vi "Review Fiducials Dialog.vi"(7 "Console Log in":refnum<class "Console Log.lvclass">, 8 "error in":errorcluster, 11 "Potting Procedure in":refnum<class "Potting Procedure.lvclass">) -> (0 "error out":errorcluster, 2 "Canceled":bool, 3 "Potting Procedure out":refnum<class "Potting Procedure.lvclass">, 5 "Console Log out":refnum<class "Console Log.lvclass">)   [LabVIEW 2011]
uses:
  Procedure Classes/Potting Procedure/Potting Procedure.lvclass
  Application Utilities/Console Log/Console Log.lvclass
  Shared Components/Utils/Type Definitions/Fiducial with Source.ctl
  Shared Components/Vec3d Class/Vec3d Class.lvclass
  Shared Components/WorkTable Class/Type Definitions/Worktable_Mode.ctl
  Procedure Classes/Potting Procedure/Type Definitions/Inspect Fiducials.ctl
  Shared Components/Utils/Type Definitions/Fiducial Image.ctl
  Shared Components/Utils/Type Definitions/Physical Image.ctl
  <vilib>/vision/Image Controls.llb/IMAQ Image.ctl
  Procedure Classes/Potting Procedure/Type Definitions/Review Fiducials.ctl
panel:
  in  "reacquire BBM BR":bool
  in  "reacquire BBM TR":bool
  in  "reacquire BBM BL":bool
  in  "reacquire BBM TL":bool
  in  "reacquire HDI BR":bool
  in  "reacquire HDI TR":bool
  in  "reacquire HDI BL":bool
  in  "reacquire HDI TL":bool
  out "BBM BL View":T1(plugin-control)
  out "BBM BR View":T1(plugin-control)
  out "BBM TL View":T1(plugin-control)
  out "BBM TR View":T1(plugin-control)
  in  "idx":i32
  out "idx_label":string="1/10"
  out "Current Module":cluster{"Chuck":i32, "Slot":i32}={"Chuck"=1, "Slot"=1}
  in  "Previous":bool
  in  "Next":bool
  out "HDI BL View":T1(plugin-control)
  out "HDI BR View":T1(plugin-control)
  out "HDI TL View":T1(plugin-control)
  out "HDI TR View":T1(plugin-control)
  in  "OK Button":bool
  in  "Cancel Button":bool
  # "Pattern Recognition"
  # "Error"
  # "Click on images to correct fiducial positions.\nAll error fiducials must be corrected before continuing."
  # "User Defined"
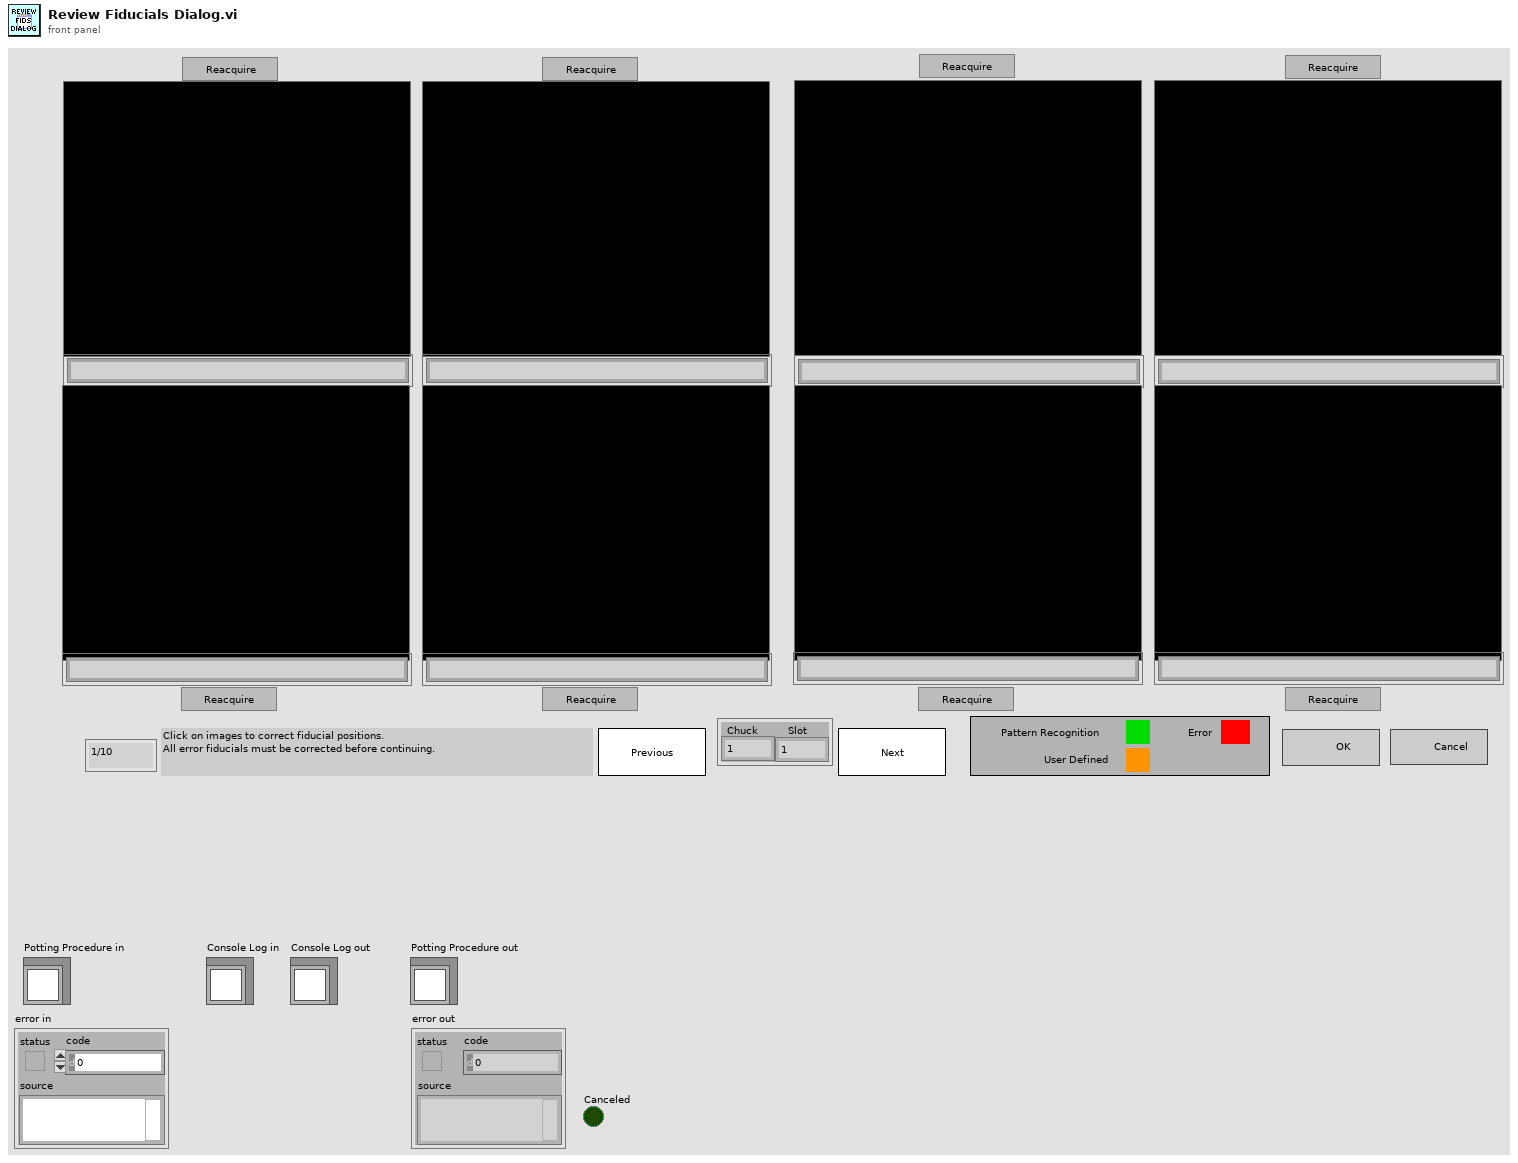
[diagram p1: front panel]
types:
  T1 = typedef "IMAQ Image.ctl" = refnum<image>
  T2 = typedef "Inspect Fiducials.ctl" = cluster{"Has Been Run?":bool, "Module-Chuck Fiducials":cluster{"Fiducials-HDI":T3[], "Fiducials-BBM":T3[], "Chuck":i32, "Slot":i32}[]}
  T3 = typedef "Fiducial Image.ctl" = cluster{"Fiducial Image":T4, "Selected Fiducial":T5, "fiducial name":string}
  T4 = typedef "Physical Image.ctl" = cluster{"Image Position":refnum<class "Vec3d Class.lvclass">, "Image Reference":T1, "Field of View":cluster{"x(mm)":dbl, "y(mm)":dbl}}
  T5 = typedef "Fiducial with Source.ctl" = cluster{"Fiducial Image Coordinate":refnum<class "Vec3d Class.lvclass">, "Fiducial Source":enum16{"Pattern Recognition", "User", "Error", "Default"}}
  T6 = cluster{"Fiducials-HDI":T3[], "Fiducials-BBM":T3[], "Chuck":i32, "Slot":i32}[]
  T7 = enum16{"None", "glue_resevoir_chuck", "stamp_tool_chuck", "weight_tool_chuck", "hdi_chuck_04"}
  T8 = typedef "Worktable_Mode.ctl" = enum16{"Encapsulation", "Gluing"}
  T9 = cluster{"Fiducials-HDI":T3[], "Fiducials-BBM":T3[], "Chuck":i32, "Slot":i32}
  T10 = enum16{"Pattern Recognition", "User", "Error", "Default"}
  T11 = typedef "LVPoint32TypeDef.ctl" = cluster{"Horizontal":i32, "Vertical":i32}
  T12 = typedef "Review Fiducials.ctl" = cluster{"Has Been Run?":bool}
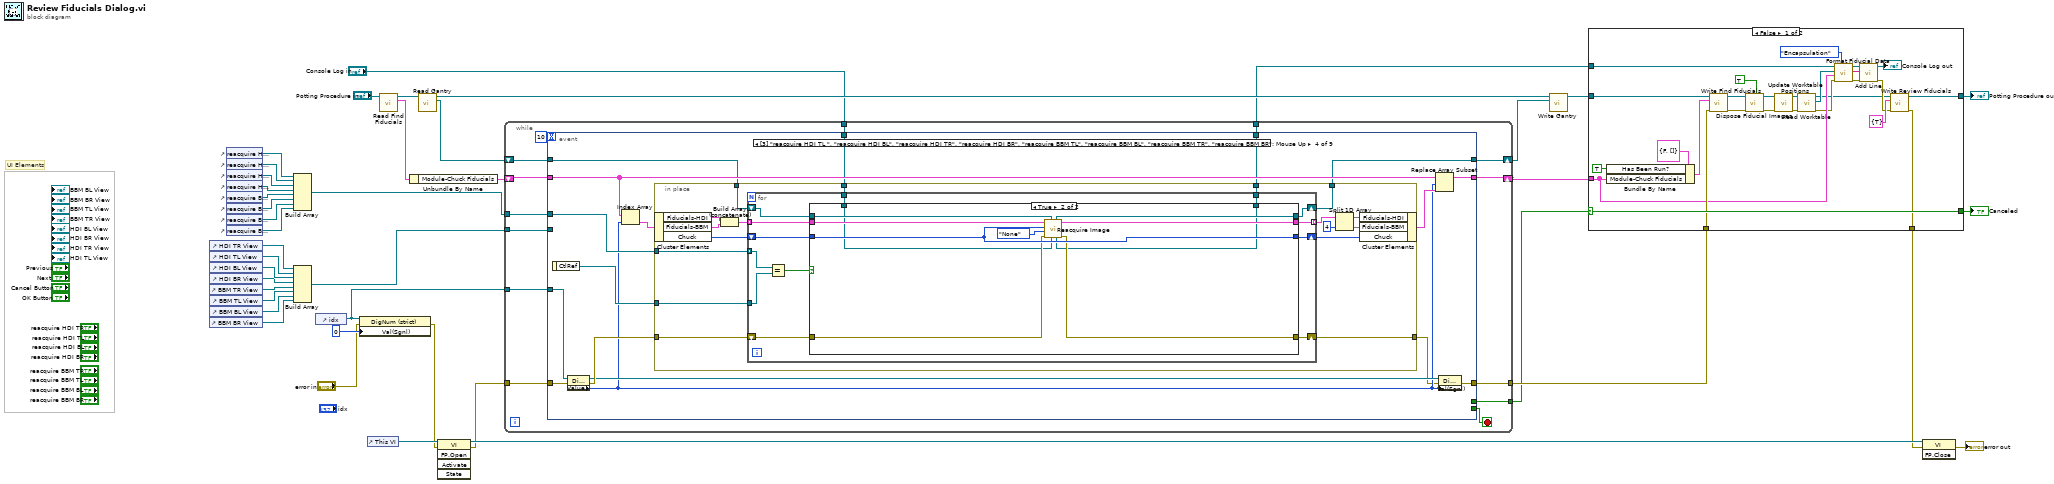
[diagram p0: block diagram]
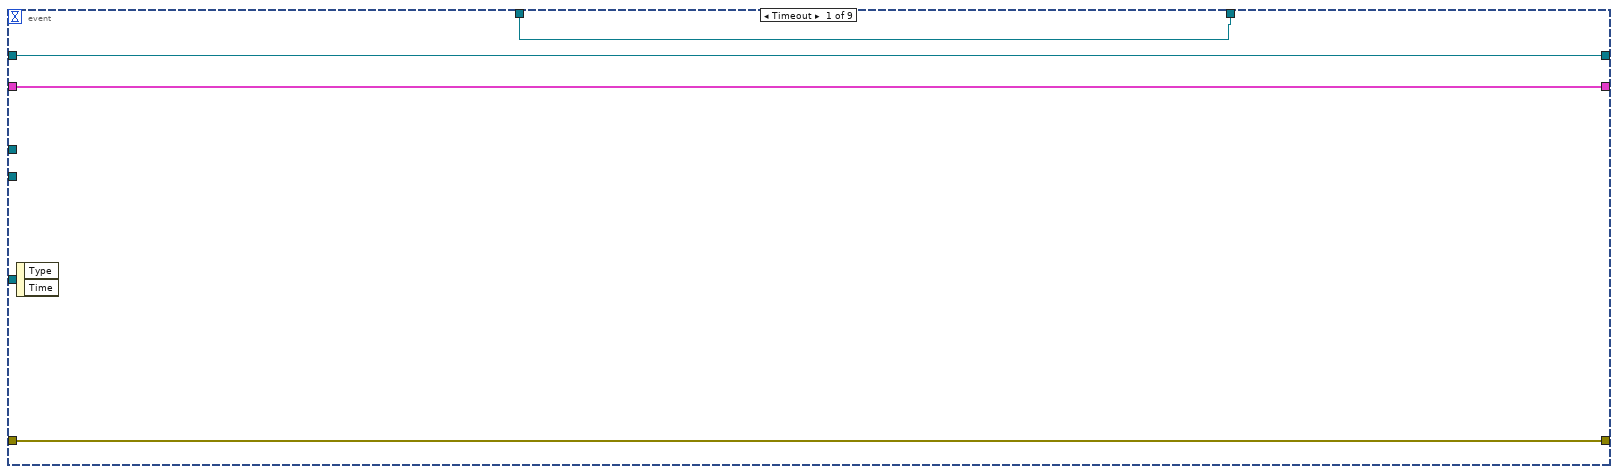
[diagram p3: hidden frame]
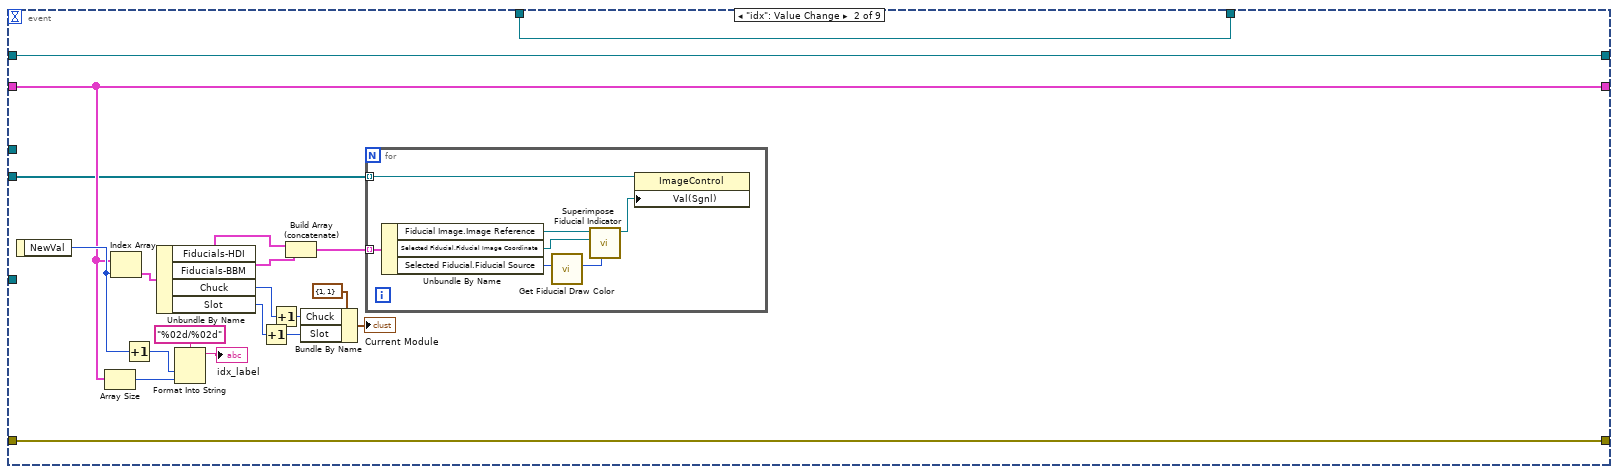
[diagram p4: hidden frame]
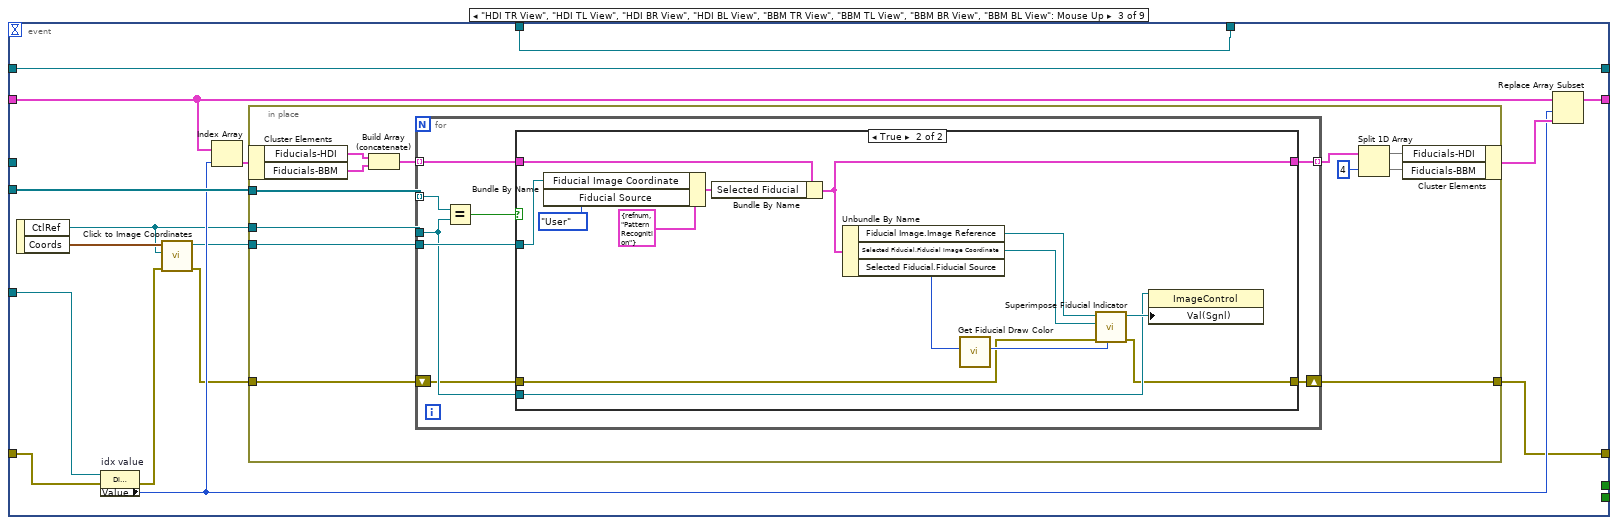
[diagram p5: hidden frame]
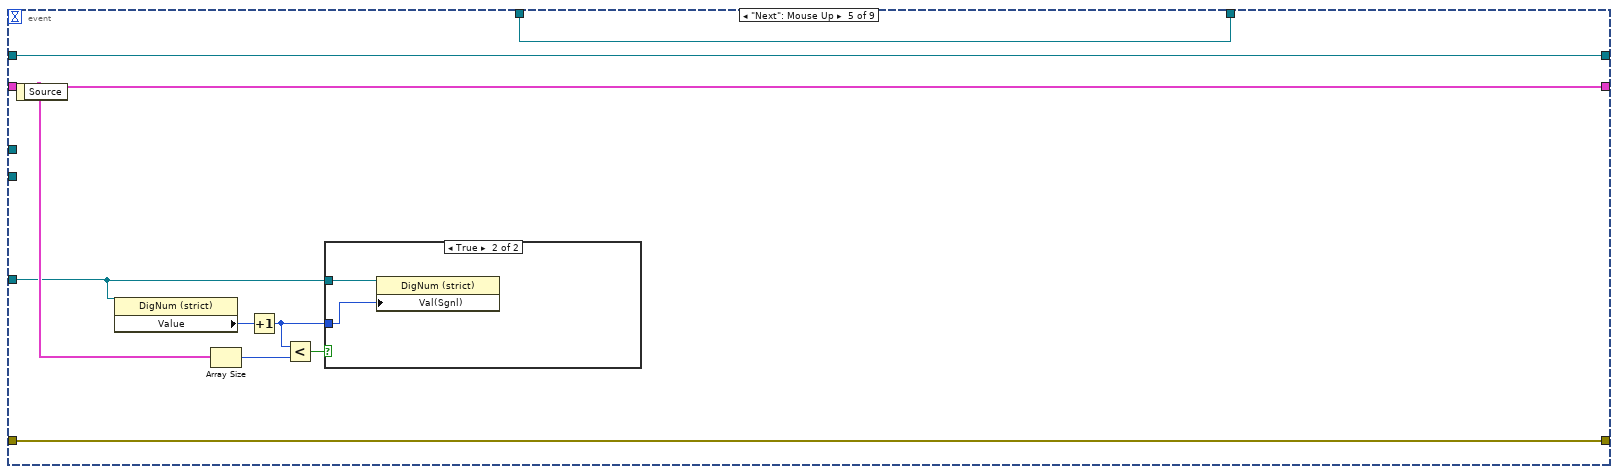
[diagram p8: hidden frame]
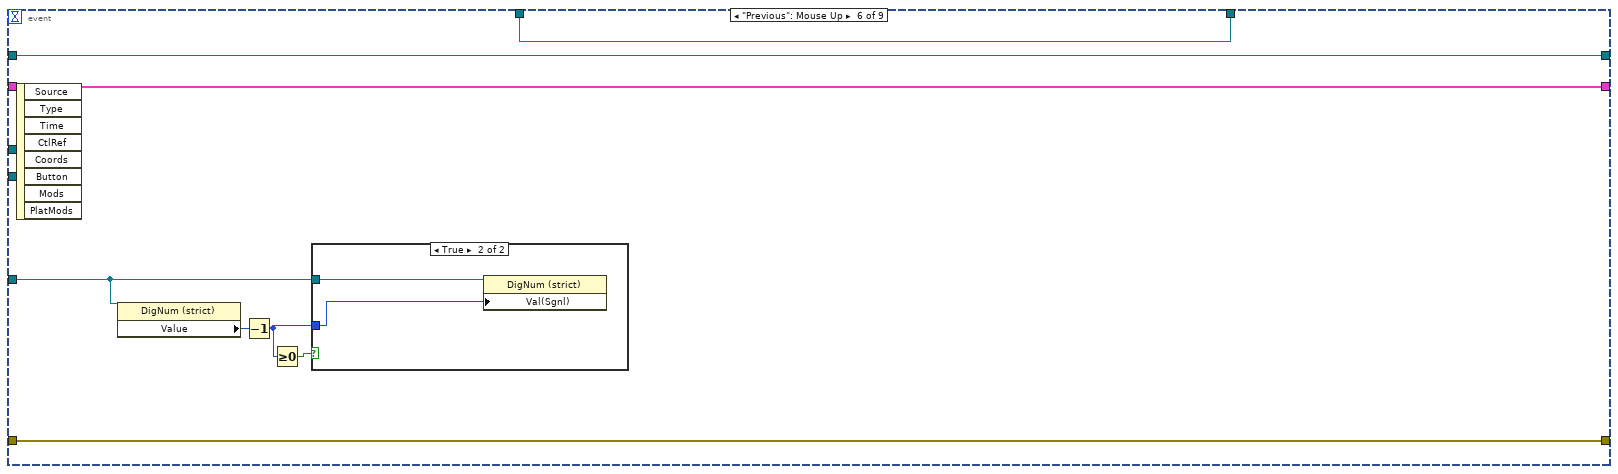
[diagram p10: hidden frame]
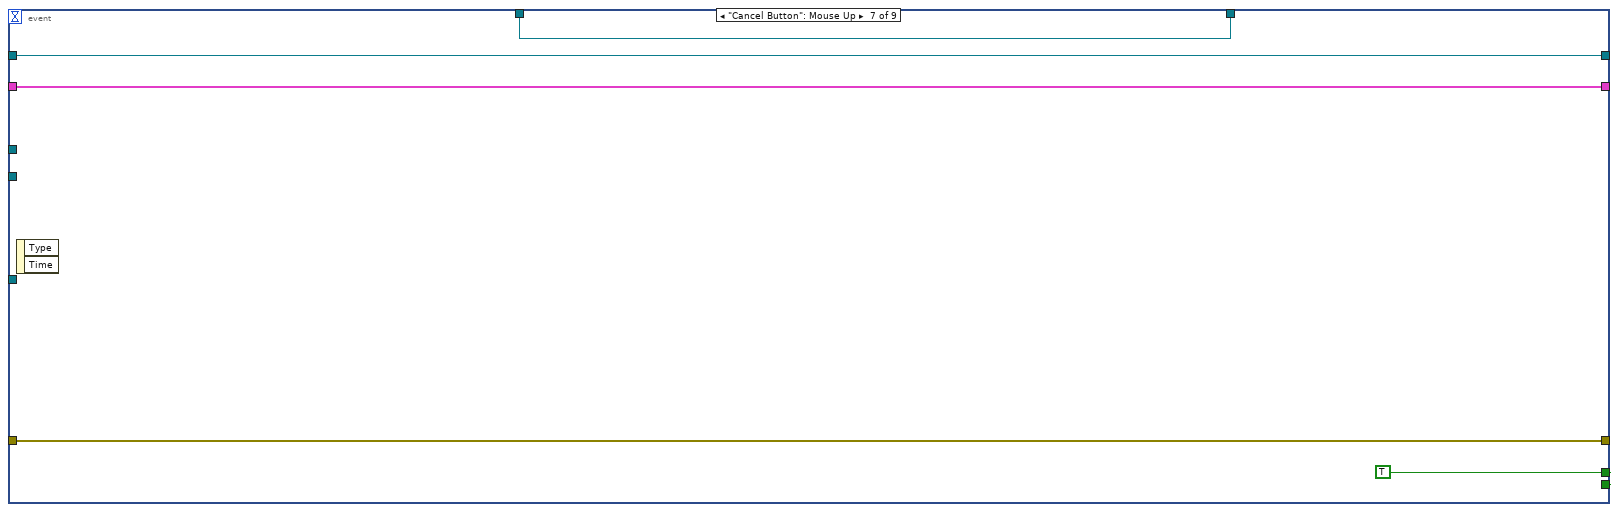
[diagram p12: hidden frame]
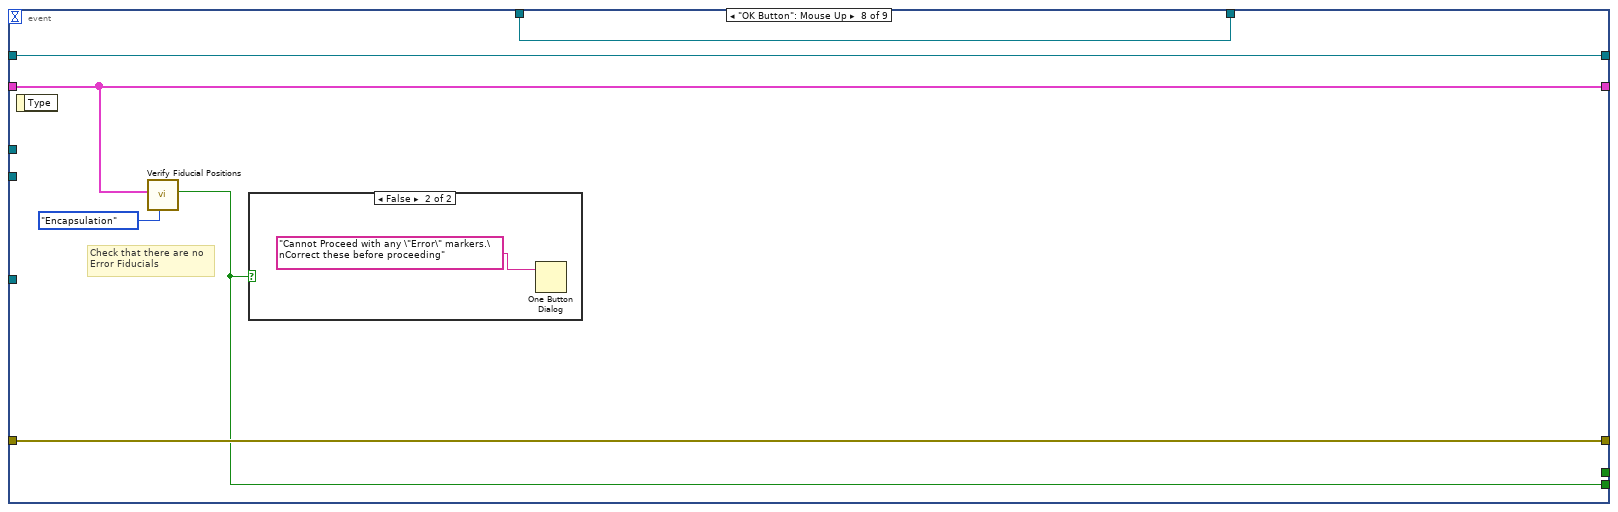
[diagram p13: hidden frame]
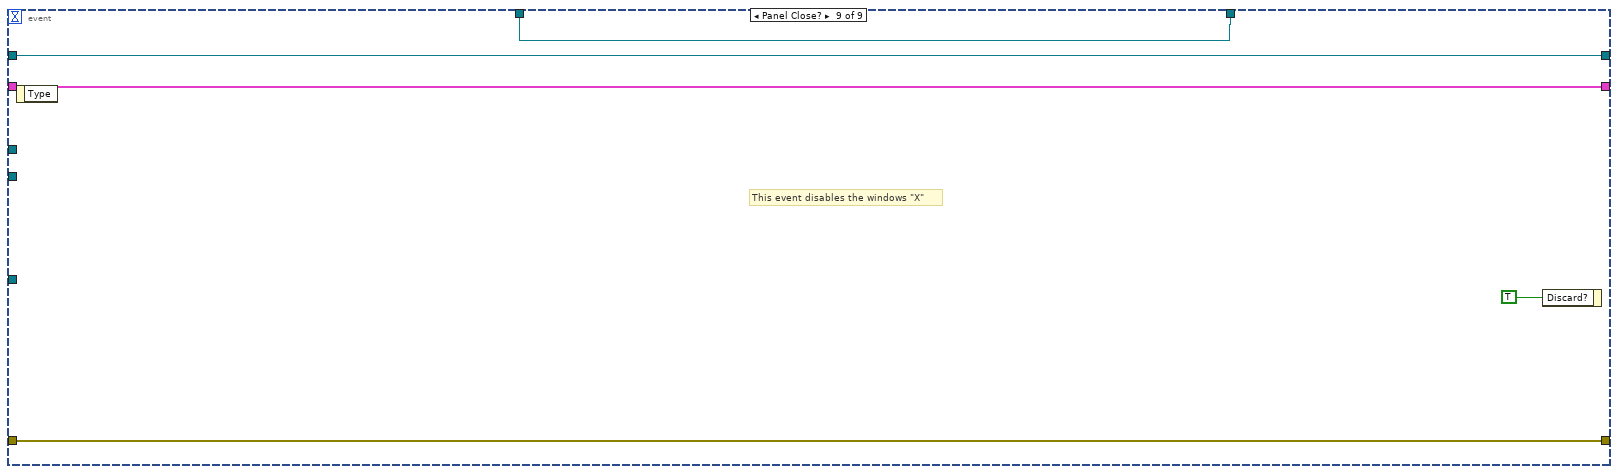
[diagram p15: hidden frame]
diagram:
  # "UI Elements"
  n1 = control-ref of="HDI TR View"() -> (w35:refnum<vi>)
  n2 = control-ref of="HDI TL View"() -> (w34:refnum<vi>)
  n3 = control-ref of="HDI BL View"() -> (w33:refnum<vi>)
  n4 = control-ref of="HDI BR View"() -> (w32:refnum<vi>)
  n5 = control-ref of="BBM TR View"() -> (w31:refnum<vi>)
  n6 = control-ref of="BBM TL View"() -> (w30:refnum<vi>)
  n7 = control-ref of="BBM BL View"() -> (w29:refnum<vi>)
  n8 = control-ref of="BBM BR View"() -> (w28:refnum<vi>)
  n9 = control-ref of="reacquire HDI TR"() -> (w9:refnum<vi>)
  n10 = control-ref of="reacquire HDI TL"() -> (w10:refnum<vi>)
  n11 = control-ref of="reacquire HDI BL"() -> (w11:refnum<vi>)
  n12 = control-ref of="reacquire HDI BR"() -> (w12:refnum<vi>)
  n13 = control-ref of="reacquire BBM TR"() -> (w13:refnum<vi>)
  n14 = control-ref of="reacquire BBM TL"() -> (w14:refnum<vi>)
  n15 = control-ref of="reacquire BBM BL"() -> (w15:refnum<vi>)
  n16 = control-ref of="reacquire BBM BR"() -> (w16:refnum<vi>)
  n17 = Build Array(w9, w10, w11, w12, w13, w14, w15, w16) -> (w8:refnum<vi>[])
  n18 = Build Array(w35, w34, w33, w32, w31, w30, w29, w28) -> (w27:refnum<vi>[])
  n19 = control-ref of="idx"() -> (w17:refnum<vi>)
  n20 = property class="DigNum (strict)"(reference=w17, error in="error in", "Val(Sgnl)"=0 ("Value (Signaling)")) -> (error out=w24:errorcluster)  [unwired: 1 out]
  n21 = control-ref of="This VI"() -> (w42:refnum<vi>)
  n22 = call-dynamic "Read Find Fiducials.vi"("Potting Procedure in"="Potting Procedure in") -> ("Find Fiducials"=w37:T2, "Potting Procedure out"=w7:refnum<class "Potting Procedure.lvclass">)  [unwired: 8 in, 1 out]
  n23 = Unbundle By Name(w37) -> ("Module-Chuck Fiducials"=w36:T6)
  n24 = call-dynamic "Read Gantry.vi"("Potting Procedure in"=w7) -> ("Gantry"=w6:refnum<class "Gantry Class.lvclass">, "Potting Procedure out"=w4:refnum<class "Potting Procedure.lvclass">)  [unwired: 8 in, 1 out]
  n25 = invoke class="VI" method="FP.Open"(reference=w42, error in=w24) -> (reference out=w41:refnum<vi>, error out=w39:errorcluster)  [unwired: 3 in, 3 out]
  n26 = while {
    tunnel: [w52] -> w22
    tunnel: w39 -> [w53]
    tunnel: [w54] -> w23
    shift-right: [w51] -> w21
    shift-left: w36 -> [w50]
    tunnel: w27 -> [w49]
    tunnel: w17 -> [w48]
    tunnel: w8 -> [w47]
    shift-right: [w45] -> w3
    shift-left: w6 -> [w46]
    tunnel: "Console Log in" -> [w44]
    tunnel: [w43] -> w1
    stop <- w55 stop-if-true
    n27 = event shown="[3] \"reacquire HDI TL \", \"reacquire HDI BL\", \"reacquire HDI TR\", \"reacquire HDI BR\", \"reacquire BBM TL\", \"reacquire BBM BL\", \"reacquire BBM TR\", \"reacquire BBM BR\": Mouse Up" {
      selector: _ -> [_ _ _ _ _ _ _ _ _]
      dyn-events: _ -> [_ _ _ _ _ _ _ _ _]
      timeout: 10 -> [_ _ _ _ _ _ _ _ _]
      tunnel: [_ _ _ _ _ _ w226 w231 _] -> w55
      tunnel: [w60 w63 w90 w145 w204 w215 w227 w233 w238] -> w54
      tunnel: w53 -> [w60 w63 w93 w155 w204 w215 w227 w233 w238]
      tunnel: [_ _ _ _ _ _ w226 _ _] -> w52
      tunnel: [w59 w72 w101 w150 w206 w217 w225 w232 w237] -> w51
      tunnel: w50 -> [w59 w72 w102 w151 w206 w217 w225 w232 w237]
      tunnel: w49 -> [_ w69 w103 _ _ _ _ _ _]
      tunnel: w48 -> [_ _ w97 w156 w205 w216 _ _ _]
      tunnel: w47 -> [_ _ _ w153 _ _ _ _ _]
      tunnel: w46 -> [w58 w62 w89 w143 w203 w214 w224 w230 w236]
      tunnel: [w58 w62 w89 w142 w203 w214 w224 w230 w236] -> w45
      tunnel: w44 -> [w57 w61 w88 w141 w202 w213 w223 w229 w235]
      tunnel: [w57 w61 w88 w140 w202 w213 w223 w229 w235] -> w43
      event Timeout {
        n28 = event-data() -> ()  [unwired: 1 in, 2 out]
      }
      event "idx": Value Change {
        n29 = event-data() -> ("NewVal"=w74:i32)  [unwired: 1 in]
        n30 = Array Size(array=w72) -> (size(s)=w75:i32)
        n31 = Index Array(array=w72, index=w74) -> (element=w80:T9)
        n32 = Increment(x=w74) -> (x+1=w76:i32)
        n33 = Unbundle By Name(w80) -> ("Fiducials-HDI"=w70:T3[], "Fiducials-BBM"=w71:T3[], "Chuck"=w64:i32, "Slot"=w66:i32)
        n34 = Format Into String(format string="%02d/%02d", w76, w75) -> (resulting string=→"idx_label":string)  [unwired: 2 in, 1 out]
        n35 = Increment(x=w66) -> (x+1=w67:i32)
        n36 = Increment(x=w64) -> (x+1=w65:i32)
        n37 = Build Array (concatenate)(w70, w71) -> (w68:T3[])
        n38 = Bundle By Name(cluster=cluster{"Chuck":i32, "Slot":i32} {"Chuck"=1, "Slot"=1} ("Current Module"), "Chuck"=w65, "Slot"=w67) -> (→"Current Module":cluster{"Chuck":i32, "Slot":i32})
        n39 = for {
          tunnel: w69 -> [w86] mode=indexing
          tunnel: w68 -> [w87] mode=indexing
          n40 = Unbundle By Name(w87) -> ("Fiducial Image.Image Reference"=w85:T1, "Selected Fiducial.Fiducial Image Coordinate"=w83:refnum<class "Vec3d Class.lvclass">, "Selected Fiducial.Fiducial Source"=w82:T10)
          n41 = call "Get Fiducial Draw Color.vi"("Fiducial Source"=w82) -> ("Grid Line Color"=w81:u32)  [unwired: 10 in]
          n42 = call "Superimpose Fiducial Indicator.vi"("Marker Color"=w81, "Fiducial Image Coordinates"=w83, "Image In"=w85) -> ("Image Out"=w84:T1)  [unwired: 7 in, 1 out]
          n43 = property class="ImageControl"(reference=w86, "Val(Sgnl)"=w84) -> ()  [unwired: 1 in, 2 out]
        }
      }
      event "HDI TR View", "HDI TL View", "HDI BR View", "HDI BL View", "BBM TR View", "BBM TL View", "BBM BR View", "BBM BL View": Mouse Up {
        n44 = event-data() -> ("CtlRef"=w94:refnum<vi>, "Coords"=w95:T11)  [unwired: 1 in]
        n45 = property on="idx value" class="DigNum (strict)"(reference=w97, error in=w93) -> (error out=w92:errorcluster, "Value"=w98:i32)  [unwired: 1 out]
        n46 = call "Click to Image Coordinates.vi"("error in"=w92, "Display Reference"=w94, "Coords"=w95) -> ("error out"=w91:errorcluster, "Image Coordinates"=w96:refnum<class "Vec3d Class.lvclass">)  [unwired: 7 in]
        n47 = Index Array(array=w102, index=w98) -> (element=w100:T9)
        n48 = in-place {
          in-place-border: w103 -> [w115]
          in-place-border: w94 -> [w113]
          in-place-border: w96 -> [w112]
          in-place-border: w91 -> [w105]
          in-place-border: [w104] -> w90
          n49 = in-place-cluster #1(w100) -> ("Fiducials-HDI"=w111:T3[], "Fiducials-BBM"=w110:T3[])
          n50 = Build Array (concatenate)(w111, w110) -> (w114:T3[])
          n51 = for {
            tunnel: w115 -> [w121] mode=indexing
            tunnel: w114 -> [w123] mode=indexing
            tunnel: w113 -> [w118]
            tunnel: w112 -> [w120]
            tunnel: [w119] -> w109 mode=indexing
            shift-right: [w116] -> w104
            shift-left: w105 -> [w117]
            n52 = Equal?(x=w121, y=w118) -> (x = y?=w122:bool)
            n53 = case shown="True" w122 {
              tunnel: w123 -> [w125 w135]
              tunnel: w120 -> [_ w138]
              tunnel: [w125 w131] -> w119
              tunnel: w118 -> [_ w130]
              tunnel: w117 -> [w124 w127]
              tunnel: [w124 w126] -> w116
              frame False {
              }
              frame True {
                n54 = Bundle By Name(cluster=T5 {"Fiducial Image Coordinate"=refnum, "Fiducial Source"=enum."Pattern Recognition"} ("Selected Fiducial"), "Fiducial Image Coordinate"=w138, "Fiducial Source"=enum16{"Pattern Recognition", "User", "Error"}."User") -> (w136:T5)
                n55 = Bundle By Name(cluster=w135, "Selected Fiducial"=w136) -> (w131:T3)
                n56 = Unbundle By Name(w131) -> ("Fiducial Image.Image Reference"=w133:T1, "Selected Fiducial.Fiducial Image Coordinate"=w132:refnum<class "Vec3d Class.lvclass">, "Selected Fiducial.Fiducial Source"=w129:T10)
                n57 = call "Get Fiducial Draw Color.vi"("Fiducial Source"=w129) -> ("Grid Line Color"=w128:u32)  [unwired: 10 in]
                n58 = call "Superimpose Fiducial Indicator.vi"("Marker Color"=w128, "error in"=w127, "Fiducial Image Coordinates"=w132, "Image In"=w133) -> ("error out"=w126:errorcluster, "Image Out"=w134:T1)  [unwired: 6 in]
                n59 = property class="ImageControl"(reference=w130, "Val(Sgnl)"=w134) -> ()  [unwired: 1 in, 2 out]
              }
            }
          }
          n60 = Split 1D Array(array=w109, index=4) -> (first subarray=w108:T3[], second subarray=w107:T3[])
          n61 = in-place-cluster #1("Fiducials-HDI"=w108, "Fiducials-BBM"=w107) -> (w99:T9)
        }
        n62 = Replace Array Subset(array=w102, new element=w99, index=w98) -> (w101:T6)
      }
      event "reacquire HDI TL", "reacquire HDI BL", "reacquire HDI TR", "reacquire HDI BR", "reacquire BBM TL", "reacquire BBM BL", "reacquire BBM TR", "reacquire BBM BR": Mouse Up {
        n63 = event-data() -> ("CtlRef"=w154:refnum<vi>)  [unwired: 1 in]
        n64 = property class="DigNum (strict)"(reference=w156, error in=w155) -> (reference out=w147:refnum<vi>, error out=w148:errorcluster, "Value"=w146:i32)
        n65 = Index Array(array=w151, index=w146) -> (element=w152:T9)
        n66 = in-place {
          in-place-border: w154 -> [w172]
          in-place-border: w153 -> [w171]
          in-place-border: w148 -> [w164]
          in-place-border: [w163] -> w144
          in-place-border: w143 -> [w160]
          in-place-border: [w159] -> w142
          in-place-border: w141 -> [w158]
          in-place-border: [w157] -> w140
          n67 = in-place-cluster #2(w152) -> ("Fiducials-HDI"=w169:T3[], "Fiducials-BBM"=w170:T3[], "Chuck"=w162:i32)
          n68 = Build Array (concatenate)(w169, w170) -> (w173:T3[])
          n69 = for {
            tunnel: w173 -> [w184] mode=indexing
            tunnel: w172 -> [w185]
            tunnel: w171 -> [w186] mode=indexing
            tunnel: [w182] -> w167 mode=indexing
            shift-right: [w180] -> w163
            shift-left: w164 -> [w181]
            shift-right: [w179] -> w161
            shift-left: w162 -> [w178]
            tunnel: w158 -> [w175]
            tunnel: [w174] -> w157
            shift-right: [w176] -> w159
            shift-left: w160 -> [w177]
            n70 = Equal?(x=w186, y=w185) -> (x = y?=w183:bool)
            n71 = case shown="True" w183 {
              tunnel: w184 -> [w191 w195]
              tunnel: [w191 w199] -> w182
              tunnel: w181 -> [w190 w197]
              tunnel: [w190 w196] -> w180
              tunnel: [w189 w198] -> w179
              tunnel: w178 -> [w189 w198]
              tunnel: w177 -> [w188 w201]
              tunnel: [w188 w200] -> w176
              tunnel: w175 -> [w187 w194]
              tunnel: [w187 w193] -> w174
              frame False {
              }
              frame True {
                n72 = call "Reacquire Image.vi"("Console Log in"=w194, "Gantry in"=w201, "error in"=w197, "Tool Chuck?"=T7."None", "Chuck"=w198, "Fiducial Image In"=w195) -> ("error out"=w196:errorcluster, "Fiducial Image Out"=w199:T3, "Console Log out"=w193:refnum<class "Console Log.lvclass">, "Gantry out"=w200:refnum<class "Gantry Class.lvclass">)  [unwired: 2 in]
              }
            }
          }
          n73 = Split 1D Array(array=w167, index=4) -> (first subarray=w166:T3[], second subarray=w165:T3[])
          n74 = in-place-cluster #2("Fiducials-HDI"=w166, "Fiducials-BBM"=w165, "Chuck"=w161) -> (w149:T9)
        }
        n75 = Replace Array Subset(array=w151, new element=w149, index=w146) -> (w150:T6)
        n76 = property class="DigNum (strict)"(reference=w147, error in=w144, "Val(Sgnl)"=w146) -> (error out=w145:errorcluster)  [unwired: 1 out]
      }
      event "Next": Mouse Up {
        n77 = event-data() -> ()  [unwired: 1 in, 1 out]
        n78 = property class="DigNum (strict)"(reference=w205) -> ("Value"=w210:i32)  [unwired: 1 in, 2 out]
        n79 = Array Size(array=w206) -> (size(s)=w209:i32)
        n80 = Increment(x=w210) -> (x+1=w207:i32)
        n81 = Less?(x=w207, y=w209) -> (x < y?=w208:bool)
        n82 = case shown="True" w208 {
          tunnel: w207 -> [_ w211]
          tunnel: w205 -> [_ w212]
          frame False {
          }
          frame True {
            n83 = property class="DigNum (strict)"(reference=w212, "Val(Sgnl)"=w211) -> ()  [unwired: 1 in, 2 out]
          }
        }
      }
      event "Previous": Mouse Up {
        n84 = event-data() -> ()  [unwired: 1 in, 8 out]
        n85 = property class="DigNum (strict)"(reference=w216) -> ("Value"=w220:i32)  [unwired: 1 in, 2 out]
        n86 = Decrement(x=w220) -> (x-1=w218:i32)
        n87 = Greater Or Equal To 0?(x=w218) -> (x >= 0?=w219:bool)
        n88 = case shown="True" w219 {
          tunnel: w218 -> [_ w221]
          tunnel: w216 -> [_ w222]
          frame False {
          }
          frame True {
            n89 = property class="DigNum (strict)"(reference=w222, "Val(Sgnl)"=w221) -> ()  [unwired: 1 in, 2 out]
          }
        }
      }
      event "Cancel Button": Mouse Up {
        w226 = TRUE
        n90 = event-data() -> ()  [unwired: 1 in, 2 out]
      }
      event "OK Button": Mouse Up {
        # "Check that there are no\nError Fiducials"
        n91 = event-data() -> ()  [unwired: 1 in, 1 out]
        n92 = call "Verify Fiducial Positions.vi"("Procedure Type"=Worktable_Mode."Encapsulation", "Module Fiducials"=w232) -> ("All Good"=w231:bool)  [unwired: 8 in, 1 out]
        n93 = case shown="False" w231 {
          frame True {
          }
          frame False {
            n94 = One Button Dialog(message="Cannot Proceed with any \"Error\" markers.\nCorrect these before proceeding") -> ()  [unwired: 1 in, 1 out]
          }
        }
      }
      event Panel Close? {
        # "This event disables the windows \"X\""
        n95 = event-data() -> ()  [unwired: 1 in, 1 out]
        n96 = event-data("Discard?"=TRUE) -> ()  [unwired: 1 in, 1 out]
      }
    }
  }
  n97 = call-dynamic "Write Gantry.vi"("Gantry"=w3, "Potting Procedure in"=w4) -> ("Potting Procedure out"=w5:refnum<class "Potting Procedure.lvclass">)  [unwired: 8 in, 1 out]
  n98 = case shown="False" w22 {
    selector: w22 -> [w266 w267]
    tunnel: w23 -> [w263 w268]
    tunnel: w21 -> [w250 _]
    tunnel: w5 -> [w258 w269]
    tunnel: [w265 w269] -> w20
    tunnel: [w262 w268] -> w19
    tunnel: [w266 w267] -> w18
    tunnel: w1 -> [w242 _]
    frame False {
      n99 = Bundle By Name(cluster=T2 {"Has Been Run?"=FALSE, "Module-Chuck Fiducials"=[]} ("Find Fiducials"), "Has Been Run?"=TRUE, "Module-Chuck Fiducials"=w250) -> (w259:T2)
      n100 = call-dynamic "Write Find Fiducials.vi"("error in"=w263, "Find Fiducials"=w259, "Potting Procedure in"=w258) -> ("error out"=w255:errorcluster, "Potting Procedure out"=w257:refnum<class "Potting Procedure.lvclass">)  [unwired: 7 in]
      n101 = call-dynamic "Dispose Fiducial Images.vi"("Archive"=TRUE, "error in"=w255, "Potting Procedure in"=w257) -> ("error out"=w254:errorcluster, "Potting Procedure out"=w256:refnum<class "Potting Procedure.lvclass">)  [unwired: 7 in]
      n102 = call-dynamic "Update Worktable Positions.vi"("error in"=w254, "Potting Procedure in"=w256) -> ("error out"=w252:errorcluster, "Potting Procedure out"=w253:refnum<class "Potting Procedure.lvclass">)  [unwired: 8 in]
      n103 = call-dynamic "Read Worktable.vi"("error in"=w252, "Potting Procedure in"=w253) -> ("error out"=w246:errorcluster, "WorkTable out"=w251:refnum<class "WorkTable Class.lvclass">, "Potting Procedure out"=w243:refnum<class "Potting Procedure.lvclass">)  [unwired: 7 in]
      n104 = call "Format Fiducial Data.vi"("Procedure Type"=Worktable_Mode."Encapsulation", "error in"=w246, "Module-Chuck Fiducials"=w250, "Worktable"=w251, "Console Log in"=w242) -> ("error out"=w245:errorcluster, "Formatted Fiducial Data"=w247:string, "Console Log out"=w249:refnum<class "Console Log.lvclass">)  [unwired: 4 in]
      n105 = call "Add Line.vi"("error in"=w245, "String"=w247, "Console Log in"=w249) -> ("error out"=w244:errorcluster, "Console Log out"=→"Console Log out":refnum<class "Console Log.lvclass">)  [unwired: 7 in]
      n106 = call-dynamic "Write Review Fiducials.vi"("error in (no error)"=w244, "Review Fiducials"=T12 {"Has Been Run?"=TRUE}, "Potting Procedure in"=w243) -> ("error out"=w262:errorcluster, "Potting Procedure out"=w265:refnum<class "Potting Procedure.lvclass">)  [unwired: 7 in]
    }
    frame True {
    }
  }
  "Canceled" <- w18
  "Potting Procedure out" <- w20
  n107 = invoke class="VI" method="FP.Close"(reference=w41, error in=w19) -> (error out=→"error out":errorcluster)  [unwired: 1 in, 2 out]
